vi "Update Mode Pin.vi"(6 "Mode Cache in":u16 format="%.0b", 8 "error in (no error)":errorcluster, 9 "Mode":T2, 10 "Pin":T3=1 min=1 max=16, 11 "Chip Address (A2 A1 A0)":T4 max=7) -> (0 "error out":errorcluster, 3 "SPI Command":T1, 4 "Mode Cache out":u16 format="%.0b")   [LabVIEW 2014, in "SLSC configuration Shared.lvlib"]
doc: "Updates the mode of a single pin on the chip. This requires knowledge of the current mode of all pins."
uses:
  SLSC configuration Shared.lvlib
  Chip Address.ctl
  Pin.ctl
  Pin Mode.ctl
  SPI Command.ctl
  IOCON BANK 0 Reg Addresses.ctl
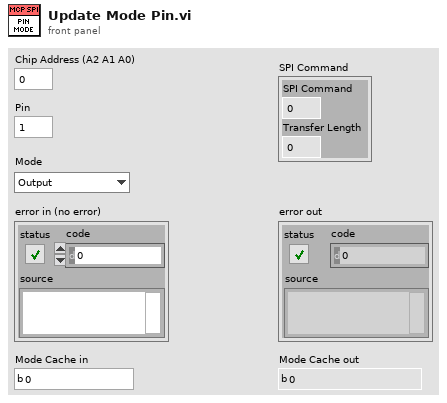
[diagram p1: front panel]
types:
  T1 = typedef "SLSC configuration Shared.lvlib/SPI Command.ctl" = cluster{"SPI Command":u32, "Transfer Length":u8}
  T2 = typedef "SLSC configuration Shared.lvlib/Pin Mode.ctl" = enum8{"Output", "Input"}
  T3 = typedef "SLSC configuration Shared.lvlib/Pin.ctl" = u8
  T4 = typedef "SLSC configuration Shared.lvlib/Chip Address.ctl" = u8
  T5 = typedef "SLSC configuration Shared.lvlib/IOCON BANK 0 Reg Addresses.ctl" = enum8{"IODIRA", "IODIRB", "IPOLA", "IPOLB", "GPINTENA", "GPINTENB", "DEFVALA", "DEFVALB", "INTCONA", "INTCONB", "IOCONA", "IOCONB", "GPPUA", "GPPUB", "INTFA", "INTFB", "INTCAPA", "INTCAPB", "GPIOA", "GPIOB", "OLATA", "OLATB"}
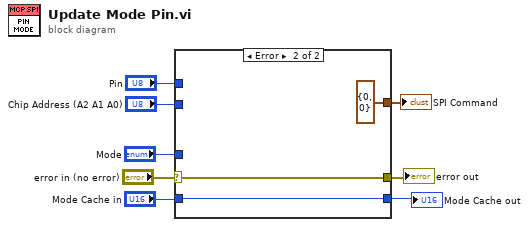
[diagram p0: block diagram]
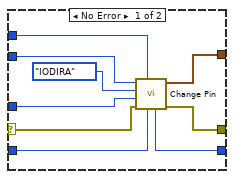
[diagram p2: hidden frame]
diagram:
  n1 = case shown="Error" "error in (no error)" {
    selector: "error in (no error)" -> [w9 w20]
    tunnel: "Chip Address (A2 A1 A0)" -> [w16 _]
    tunnel: [w15 T1 {"SPI Command"=0, "Transfer Length"=0} ("SPI Command")] -> w1
    tunnel: "Pin" -> [w10 _]
    tunnel: "Mode" -> [w11 _]
    tunnel: "Mode Cache in" -> [w14 w19]
    tunnel: [w13 w19] -> w5
    tunnel: [w12 w20] -> w3
    frame No Error {
      n2 = call "Change Pin.vi"("Cache in"=w14, "Pin"=w10, "error in (no error)"=w9, "Value"=w11, "Reg Address"=IOCON_BANK_0_Reg_Addresses."IODIRA", "Chip Address (A2 A1 A0)"=w16) -> ("error out"=w12:errorcluster, "SPI Command"=w15:T1, "Cache out"=w13:u16)  [unwired: 3 in]
    }
    frame Error {
    }
  }
  "Mode Cache out" <- w5
  "error out" <- w3
  "SPI Command" <- w1
